vi "Test Get Summary of Method With Runtime Error.vi"(8 "error in (no error)":errorcluster, 11 "Result Model Result Recording Test in":refnum<class "Result Model Result Recording Test.lvclass">) -> (0 "error out":errorcluster, 3 "Result Model Result Recording Test out":refnum<class "Result Model Result Recording Test.lvclass">)   [LabVIEW 2020, in "Result Model Result Recording Test.lvclass"]
uses:
  Result Model Result Recording Test.lvclass
  source/Core/Result/Type.ctl
  source/Core/Result/Result.lvlib
  source/Core/Result/Status.ctl
  source/Core/Result/Result.ctl
  source/User Interface/Result Model/Result Model.lvclass
  865a11a4-746d-41de-93c1-4db6b0010296.vi
panel:
  out "Summary":string
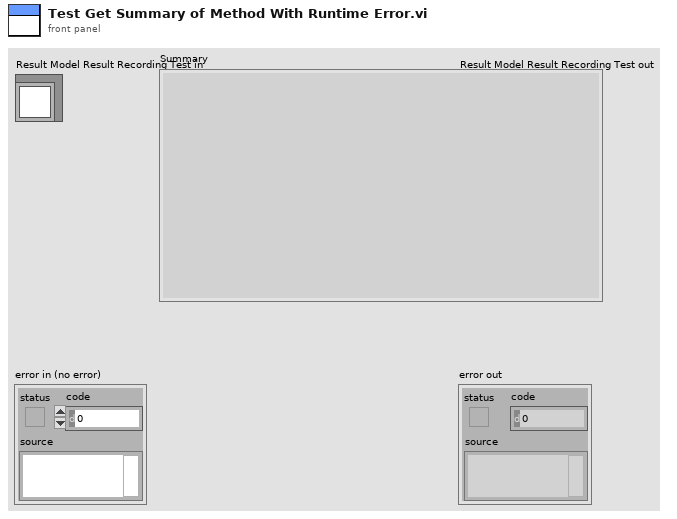
[diagram p1: front panel]
types:
  T1 = typedef "Result.lvlib/Result.ctl" = cluster{"Name":string, "Description":string, "Status":T2, "Result Type":T3, "Execution Time":dbl, "Data":cluster{"Expected":variant, "Actual":variant, "Delta":variant}}
  T2 = typedef "Result.lvlib/Status.ctl" = enum16{"", "Passed", "Failed", "Error", "Skipped", "Setup Error", "Broken", "Teardown Error"}
  T3 = typedef "Result.lvlib/Type.ctl" = enum16{"Test Case", "Test Suite", "Test Run", "Pass", "Fail", "Skip", "Pass if", "Fail if", "Pass if Error", "Fail if Error", "Pass if Equal", "Fail if Equal"}
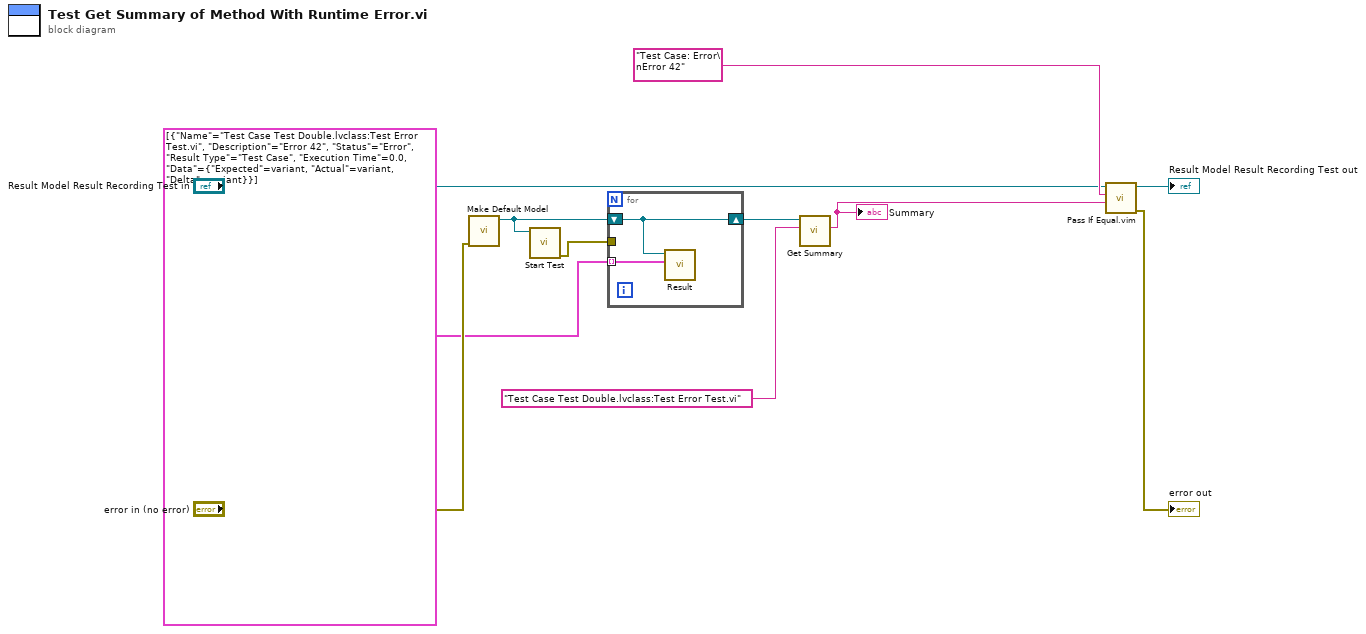
[diagram p0: block diagram]
diagram:
  n1 = call "Make Default Model.vi"("error in (no error)"="error in (no error)") -> ("Result Model out"=w2:refnum<class "Result Model.lvclass">)  [unwired: 9 in, 1 out]
  n2 = call "Start Test.vi"("Result Model by Reference In"=w2) -> ("error out"=w1:errorcluster)  [unwired: 10 in]
  n3 = for {
    tunnel: T1[] [{"Name"="Test Case Test Double.lvclass:Test Error Test.vi", "Description"="Error 42", "Status"=enum."Error", "Result Type"=enum."Test Case", "Execution Time"=0.0, "Data"={"Expected"=variant, "Actual"=variant, "Delta"=variant}}] ("Results") -> [w13] mode=indexing
    shift-right: [w12] -> w8
    shift-left: w2 -> [w12]
    tunnel: w1 -> [_]
    n4 = call-dynamic "Result.vi"("Results"=w13, "Result Model by Reference In"=w12) -> ()  [unwired: 9 in, 1 out]
  }
  n5 = call "Get Summary.vi"("Item"="Test Case Test Double.lvclass:Test Error Test.vi", "Result Model by Reference In"=w8) -> ("Summary"=w5:string)  [unwired: 8 in, 1 out]
  "Summary" <- w5
  n6 = call "Pass If Equal.vim"("Actual"=w5, "Expected"="Test Case: Error\nError 42", "LUnit Test Case In"="Result Model Result Recording Test in") -> ("error out"=→"error out":errorcluster, "LUnit Test Case Out"=→"Result Model Result Recording Test out":refnum<class "Result Model Result Recording Test.lvclass">)  [unwired: 7 in]
